vi "_PC_Pub_Dialog_XYGraphScaleSetting.vi"(7 "Function":enum16{"XScale", "YScale"}(ring)=enum."YScale", 11 "Mass spectrum":refnum<vi>) -> ()   [LabVIEW 2018]
panel:
  in  "System OK Button":bool
  in  "Maximun":dbl
  in  "Minimun":dbl
  in  "AutoScale":bool
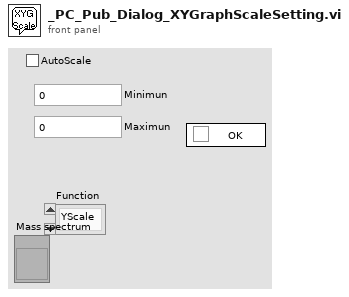
[diagram p1: front panel]
types:
  T1 = enum8{"Enabled", "Disabled", "Disabled and Grayed Out"}
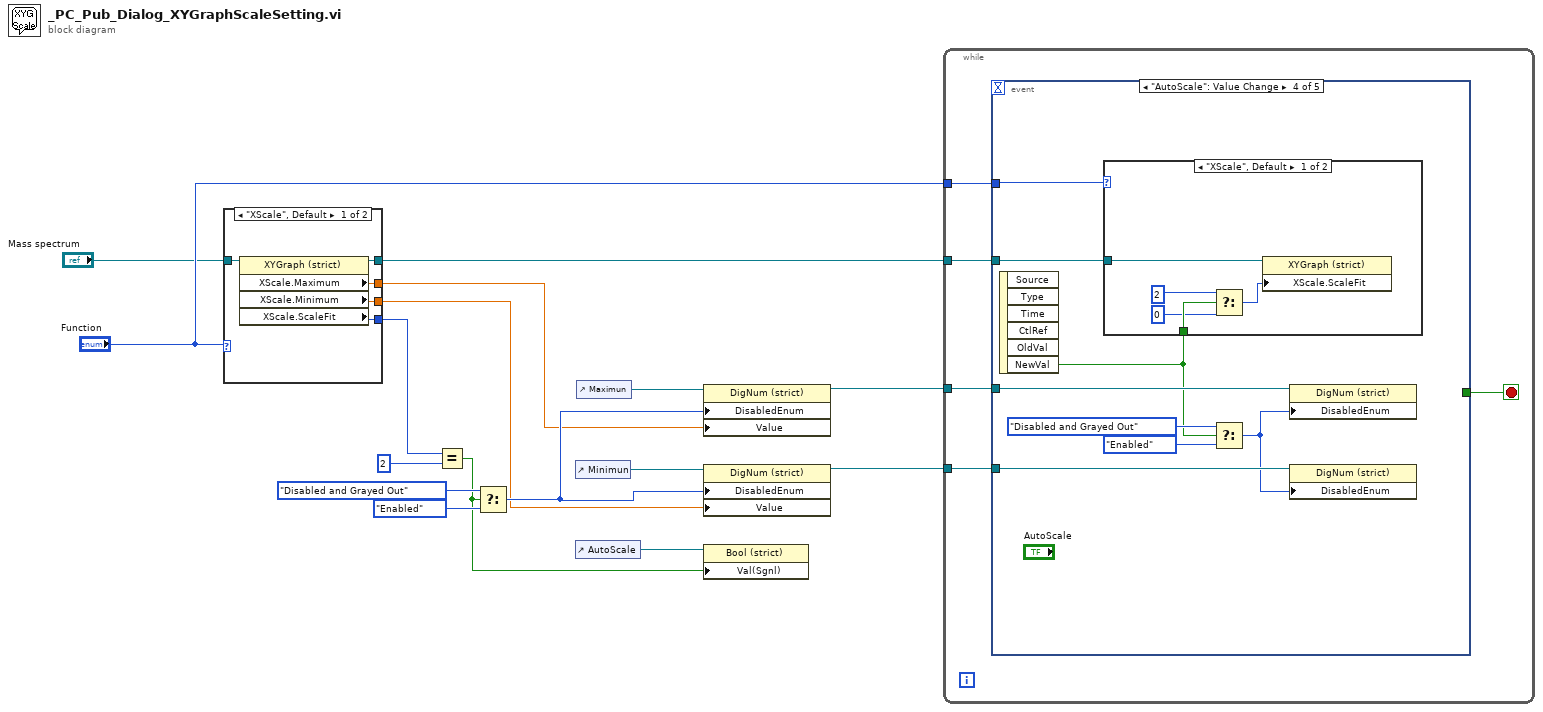
[diagram p0: block diagram]
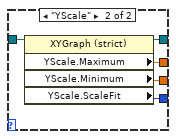
[diagram p2: hidden frame]
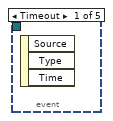
[diagram p3: hidden frame]
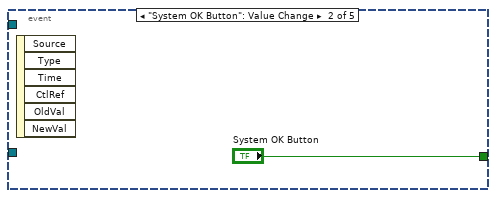
[diagram p4: hidden frame]
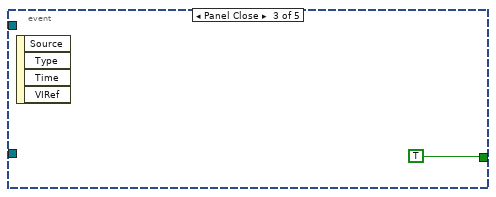
[diagram p5: hidden frame]
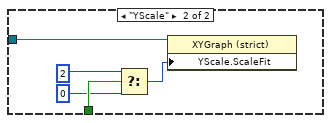
[diagram p6: hidden frame]
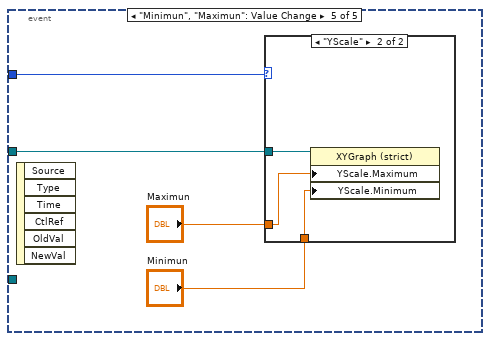
[diagram p7: hidden frame]
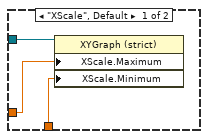
[diagram p8: hidden frame]
diagram:
  n1 = case shown="\"XScale\", Default" "Function" {
    tunnel: "Mass spectrum" -> [w21 w26]
    tunnel: [w20 w25] -> w16
    tunnel: [w19 w24] -> w9
    tunnel: [w18 w23] -> w8
    tunnel: [w17 w22] -> w3
    frame "XScale", Default {
      n2 = property class="XYGraph (strict)"(reference=w21) -> (reference out=w17:refnum<vi>, "XScale.Maximum"=w19:dbl, "XScale.Minimum"=w18:dbl, "XScale.ScaleFit"=w20:u8)  [unwired: 1 in, 1 out]
    }
    frame "YScale" {
      n3 = property class="XYGraph (strict)"(reference=w26) -> (reference out=w22:refnum<vi>, "YScale.Maximum"=w24:dbl, "YScale.Minimum"=w23:dbl, "YScale.ScaleFit"=w25:u8)  [unwired: 1 in, 1 out]
    }
  }
  n4 = Equal?(x=w16, y=u8 2) -> (x = y?=w6:bool)
  n5 = Select(t=T1."Disabled and Grayed Out" ("Disabled"), s=w6, f=T1."Enabled" ("Disabled")) -> (s? t:f=w10:T1)
  n6 = control-ref of="Minimun"() -> (w13:refnum<vi>)
  n7 = control-ref of="AutoScale"() -> (w7:refnum<vi>)
  n8 = control-ref of="Maximun"() -> (w14:refnum<vi>)
  n9 = property class="DigNum (strict)"(reference=w14, "DisabledEnum"=w10, "Value"=w9) -> (reference out=w5:refnum<vi>)  [unwired: 1 in, 1 out]
  n10 = property class="DigNum (strict)"(reference=w13, "DisabledEnum"=w10, "Value"=w8) -> (reference out=w4:refnum<vi>)  [unwired: 1 in, 1 out]
  n11 = property class="Bool (strict)"(reference=w7, "Val(Sgnl)"=w6) -> ()  [unwired: 1 in, 2 out]
  n12 = while {
    tunnel: w5 -> [w30]
    tunnel: w4 -> [w29]
    tunnel: w3 -> [w28]
    tunnel: "Function" -> [w27]
    stop <- w31 stop-if-true
    n13 = event shown="[3] \"AutoScale\": Value Change" {
      selector: _ -> [_ _ _ _ _]
      dyn-events: _ -> [_ _ _ _ _]
      timeout: _ -> [_ _ _ _ _]
      tunnel: [_ "System OK Button" TRUE _ _] -> w31
      tunnel: w30 -> [_ _ _ w41 _]
      tunnel: w29 -> [_ _ _ w40 _]
      tunnel: w28 -> [_ _ _ w36 w55]
      tunnel: w27 -> [_ _ _ w34 w52]
      event Timeout {
        n14 = event-data() -> ()  [unwired: 1 in, 3 out]
      }
      event "System OK Button": Value Change {
        n15 = event-data() -> ()  [unwired: 1 in, 6 out]
      }
      event Panel Close {
        n16 = event-data() -> ()  [unwired: 1 in, 4 out]
      }
      event "AutoScale": Value Change {
        n17 = event-data() -> ("NewVal"=w35:bool)  [unwired: 1 in, 5 out]
        n18 = case shown="\"XScale\", Default" w34 {
          tunnel: w36 -> [w46 w51]
          tunnel: w35 -> [w45 w50]
          frame "XScale", Default {
            n19 = Select(t=u8 2 ("X Scale.Scale Fit"), s=w45, f=u8 0 ("X Scale.Scale Fit")) -> (s? t:f=w42:u8)
            n20 = property class="XYGraph (strict)"(reference=w46, "XScale.ScaleFit"=w42) -> ()  [unwired: 1 in, 2 out]
          }
          frame "YScale" {
            n21 = Select(t=u8 2 ("X Scale.Scale Fit"), s=w50, f=u8 0 ("X Scale.Scale Fit")) -> (s? t:f=w47:u8)
            n22 = property class="XYGraph (strict)"(reference=w51, "YScale.ScaleFit"=w47) -> ()  [unwired: 1 in, 2 out]
          }
        }
        n23 = Select(t=T1."Disabled and Grayed Out" ("Disabled"), s=w35, f=T1."Enabled" ("Disabled")) -> (s? t:f=w37:T1)
        n24 = property class="DigNum (strict)"(reference=w41, "DisabledEnum"=w37) -> ()  [unwired: 1 in, 2 out]
        n25 = property class="DigNum (strict)"(reference=w40, "DisabledEnum"=w37) -> ()  [unwired: 1 in, 2 out]
      }
      event "Minimun", "Maximun": Value Change {
        n26 = event-data() -> ()  [unwired: 1 in, 6 out]
        n27 = case shown="\"YScale\"" w52 {
          tunnel: w55 -> [w58 w61]
          tunnel: "Maximun" -> [w57 w60]
          tunnel: "Minimun" -> [w56 w59]
          frame "XScale", Default {
            n28 = property class="XYGraph (strict)"(reference=w58, "XScale.Maximum"=w57, "XScale.Minimum"=w56) -> ()  [unwired: 1 in, 2 out]
          }
          frame "YScale" {
            n29 = property class="XYGraph (strict)"(reference=w61, "YScale.Maximum"=w60, "YScale.Minimum"=w59) -> ()  [unwired: 1 in, 2 out]
          }
        }
      }
    }
  }
